vi "Robot Arm Sally Port.vi"(7 "Start Sally Port":bool, 8 "Abort":bool, 9 "Motor Speed":dbl=-0.2, 10 "Limit Switch Elbow":bool, 11 "Limit Switch Shoulder":bool) -> (0 "Done":bool=TRUE, 1 "Arcade Drive":cluster{"x":dbl, "y":dbl}, 2 "Set Elbow":dbl, 3 "Set Shoulder":dbl, 4 "Turn Arm":bool)   [LabVIEW 2015]
uses:
  sally_port_auto_states.ctl
  Sensors.vi
panel:
  in  "Kd":dbl=0.005
  in  "Kp":dbl=0.05
  in  "Ki":dbl
  in  "Drive Time":dbl=1.1
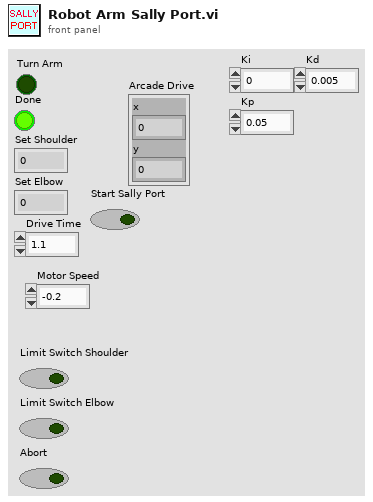
[diagram p1: front panel]
types:
  T1 = typedef "sally_port_auto_states.ctl" = enum16{"Ready", "Arm over", "Arm hook", "Arm rotate", "Move Forward for a bit", "drive thorugh", "Arm to rest", "stop"}
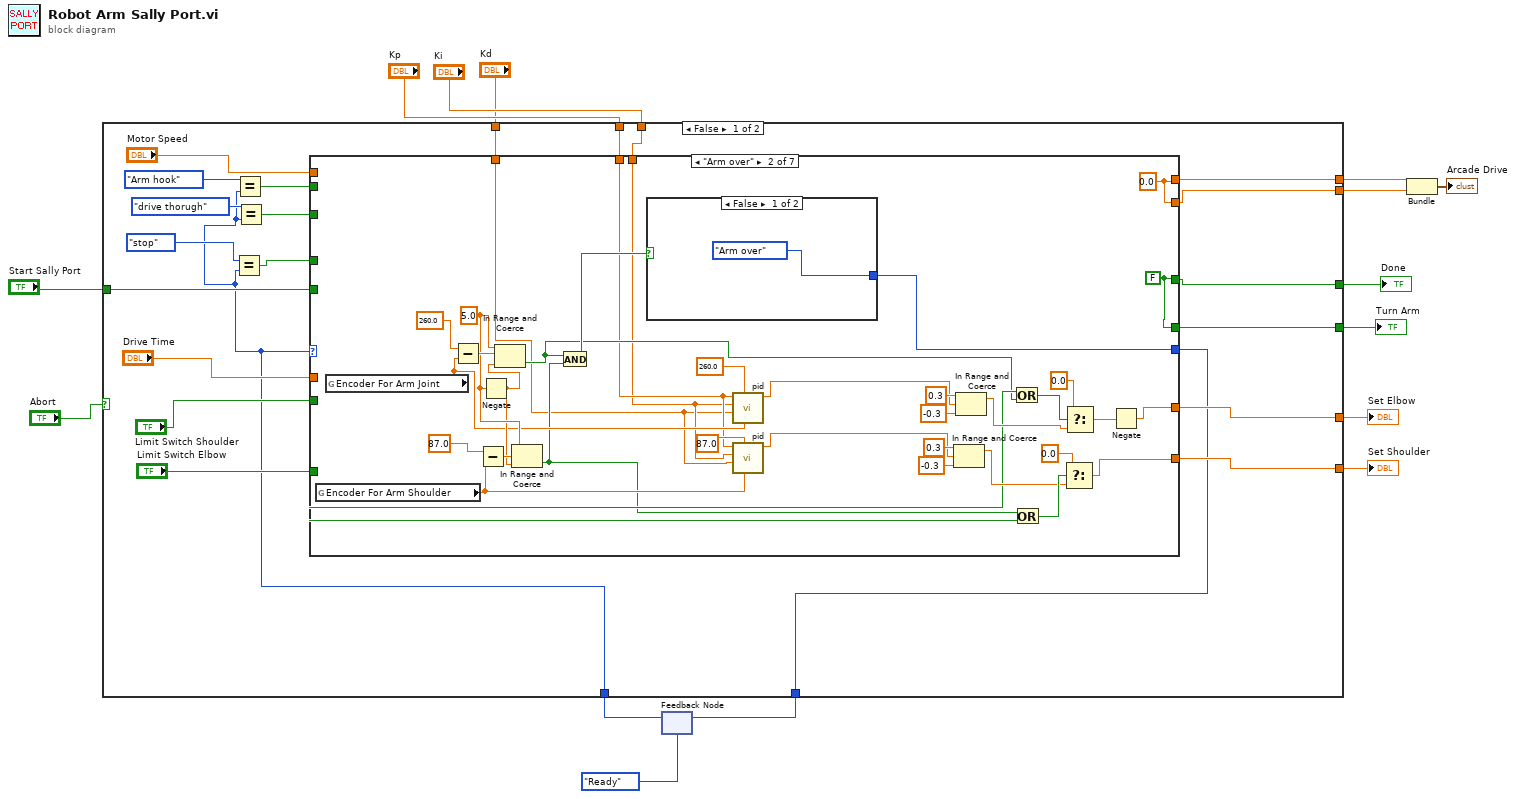
[diagram p0: block diagram]
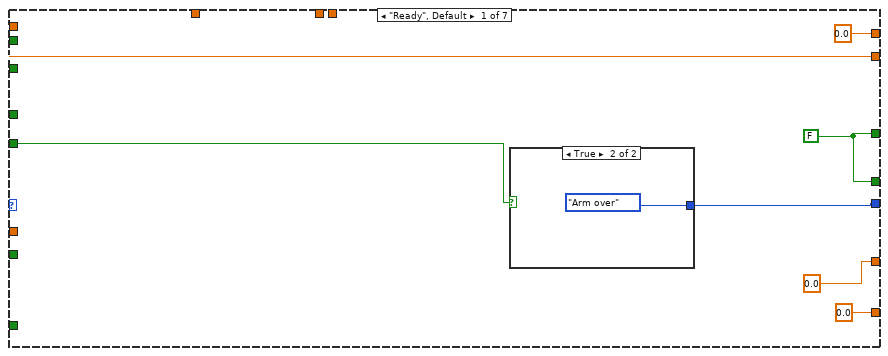
[diagram p2: hidden frame]
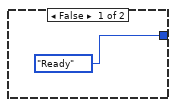
[diagram p3: hidden frame]
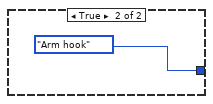
[diagram p4: hidden frame]
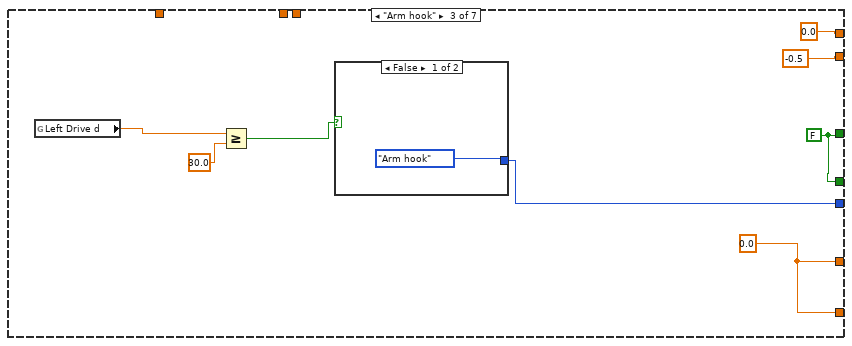
[diagram p5: hidden frame]
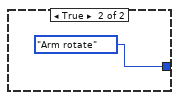
[diagram p6: hidden frame]
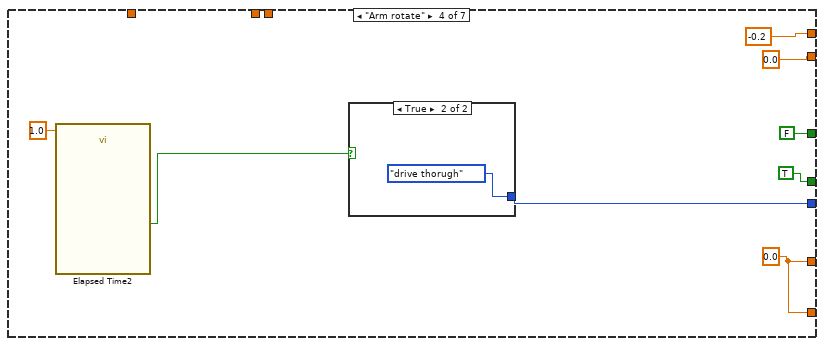
[diagram p7: hidden frame]
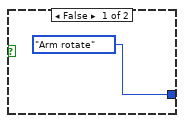
[diagram p8: hidden frame]
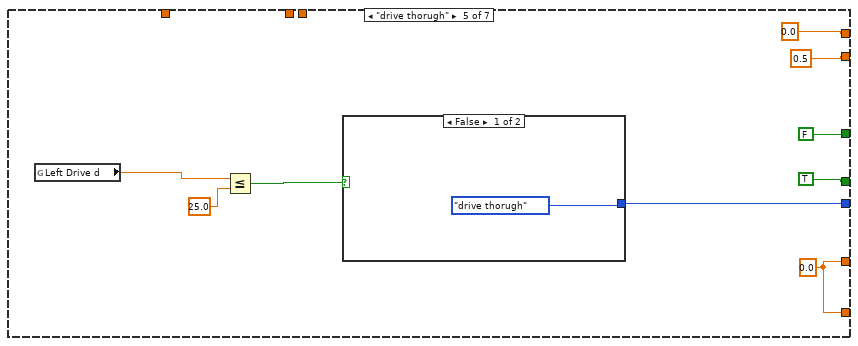
[diagram p9: hidden frame]
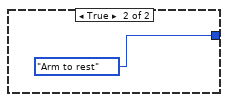
[diagram p10: hidden frame]
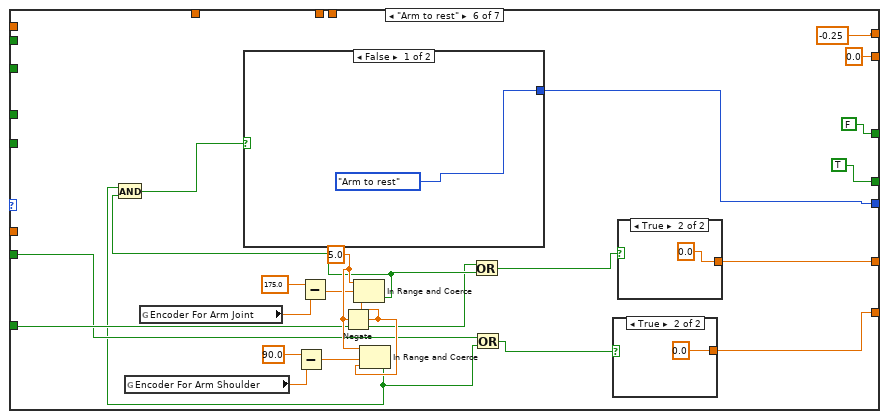
[diagram p11: hidden frame]
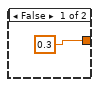
[diagram p12: hidden frame]
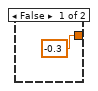
[diagram p13: hidden frame]
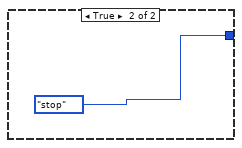
[diagram p14: hidden frame]
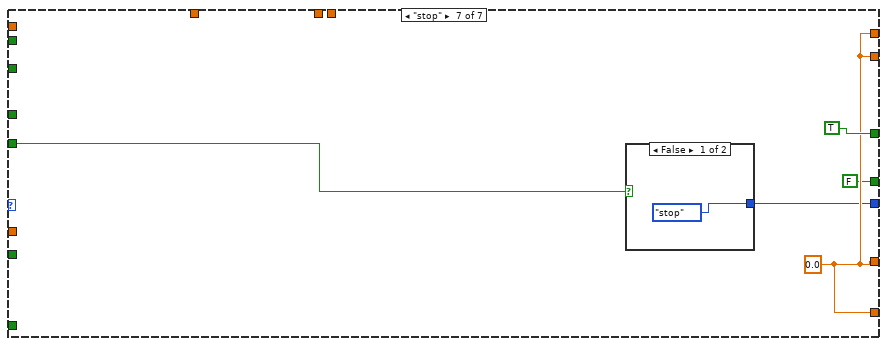
[diagram p15: hidden frame]
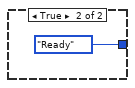
[diagram p16: hidden frame]
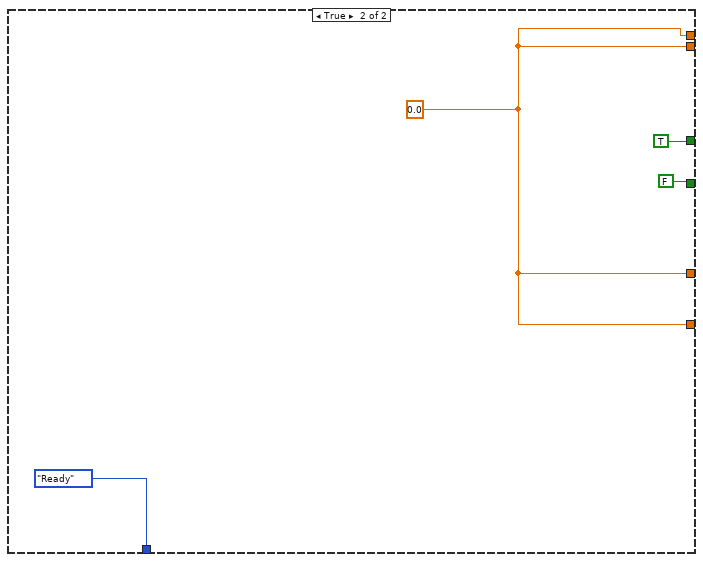
[diagram p17: hidden frame]
diagram:
  n1 = feedback #1(sally_port_auto_states."Ready") -> (w7:T1)
  n2 = case shown="False" "Abort" {
    tunnel: [w33 w154] -> w15
    tunnel: [w32 w154] -> w14
    tunnel: [w31 TRUE] -> w13
    tunnel: [w30 w154] -> w12
    tunnel: [w29 w154] -> w11
    tunnel: [w28 FALSE] -> w9
    tunnel: w7 -> [w18 _]
    tunnel: [w27 sally_port_auto_states."Ready"] -> w6
    tunnel: "Kp" -> [w26 _]
    tunnel: "Ki" -> [w25 _]
    tunnel: "Kd" -> [w24 _]
    tunnel: "Start Sally Port" -> [w23 _]
    frame False {
      n3 = Equal?(x=sally_port_auto_states."stop", y=w18) -> (x = y?=w21:bool)
      n4 = Equal?(x=sally_port_auto_states."Arm hook", y=w18) -> (x = y?=w16:bool)
      n5 = Equal?(x=sally_port_auto_states."drive thorugh", y=w18) -> (x = y?=w20:bool)
      n6 = case shown="\"Arm over\"" w18 {
        tunnel: "Motor Speed" -> [w44 _ _ _ _ _ _]
        tunnel: "Drive Time" -> [_ _ _ _ _ _ _]
        tunnel: [0.0 w71 0.0 -0.2 0.0 -0.25 w147] -> w33
        tunnel: [w38 w47 w88 FALSE FALSE FALSE TRUE] -> w31
        tunnel: [0.0 ("Set Motor at S") w56 w91 w101 w110 w134 w147] -> w30
        tunnel: [0.0 ("Set Motor at 1") w55 w91 w101 w110 w135 w147] -> w29
        tunnel: [w44 w71 -0.5 0.0 0.5 0.0 ("Motor Speed") w147] -> w32
        tunnel: "Limit Switch Shoulder" -> [_ w54 _ _ _ w120 _]
        tunnel: "Limit Switch Elbow" -> [_ w53 _ _ _ w121 _]
        tunnel: [w40 w70 w92 w102 w111 w133 w146] -> w27
        tunnel: [w38 w47 w88 TRUE TRUE TRUE FALSE] -> w28
        tunnel: w23 -> [w39 _ _ _ _ _ w144]
        tunnel: w26 -> [_ w50 _ _ _ _ _]
        tunnel: w25 -> [_ w49 _ _ _ _ _]
        tunnel: w24 -> [_ w48 _ _ _ _ _]
        tunnel: w21 -> [_ _ _ _ _ _ _]
        tunnel: w20 -> [_ _ _ _ _ _ _]
        tunnel: w16 -> [_ _ _ _ _ _ _]
        frame "Ready", Default {
          w38 = FALSE
          n7 = case shown="True" w39 {
            tunnel: [sally_port_auto_states."Ready" sally_port_auto_states."Arm over"] -> w40
            frame False {
            }
            frame True {
            }
          }
        }
        frame "Arm over" {
          w75 = 5.0
          w47 = FALSE
          w71 = 0.0
          n8 = global read "Sensors.vi" "Encoder For Arm Shoulder"() -> (w73:dbl)
          n9 = global read "Sensors.vi" "Encoder For Arm Joint"() -> (w72:dbl)
          n10 = Subtract(x=260.0 ("setpoint"), y=w72) -> (x-y=w77:dbl)
          n11 = Subtract(x=87.0 ("setpoint"), y=w73) -> (x-y=w80:dbl)
          n12 = Negate(x=w75) -> (-x=w74:dbl)
          n13 = In Range and Coerce(upper limit=w75, x=w77, lower limit=w74) -> (In Range?=w52:bool)  [unwired: 1 out]
          n14 = In Range and Coerce(upper limit=w75, x=w80, lower limit=w74) -> (In Range?=w51:bool)  [unwired: 1 out]
          n15 = And(x=w52, y=w51) -> (x .and. y?=w78:bool)
          n16 = case shown="False" w78 {
            tunnel: [sally_port_auto_states."Arm over" sally_port_auto_states."Arm hook"] -> w70
            frame False {
            }
            frame True {
            }
          }
          n17 = call "pid.vi"("y"=w72, "setpoint"=260.0, "kd"=w48, "ki"=w49, "kp"=w50) -> ("Motor Command"=w61:dbl)  [unwired: 6 in]
          n18 = call "pid.vi"("y"=w73, "setpoint"=87.0, "kd"=w48, "ki"=w49, "kp"=w50) -> ("Motor Command"=w60:dbl)  [unwired: 6 in]
          n19 = In Range and Coerce(upper limit=0.3, x=w60, lower limit=-0.3) -> (coerced(x)=w59:dbl)  [unwired: 1 out]
          n20 = In Range and Coerce(upper limit=0.3, x=w61, lower limit=-0.3) -> (coerced(x)=w58:dbl)  [unwired: 1 out]
          n21 = Or(x=w53, y=w52) -> (x .or. y?=w62:bool)
          n22 = Or(x=w51, y=w54) -> (x .or. y?=w63:bool)
          n23 = Select(t=0.0, s=w63, f=w59) -> (s? t:f=w55:dbl)
          n24 = Select(t=0.0, s=w62, f=w58) -> (s? t:f=w57:dbl)
          n25 = Negate(x=w57) -> (-x=w56:dbl)
        }
        frame "Arm hook" {
          w91 = 0.0
          w88 = FALSE
          n26 = global read "Sensors.vi" "Left Drive d"() -> (w85:dbl)
          n27 = Greater Or Equal?(x=w85, y=30.0) -> (x >= y?=w86:bool)
          n28 = case shown="False" w86 {
            tunnel: [sally_port_auto_states."Arm hook" sally_port_auto_states."Arm rotate"] -> w92
            frame False {
            }
            frame True {
            }
          }
        }
        frame "Arm rotate" {
          w101 = 0.0
          n29 = call "Elapsed Time2"("Time Target (s)"=1.0) -> ("Time has Elapsed"=w98:bool)  [unwired: 11 in, 7 out]
          n30 = case shown="True" w98 {
            tunnel: [sally_port_auto_states."Arm rotate" sally_port_auto_states."drive thorugh"] -> w102
            frame False {
            }
            frame True {
            }
          }
        }
        frame "drive thorugh" {
          w110 = 0.0
          n31 = global read "Sensors.vi" "Left Drive d"() -> (w106:dbl)
          n32 = Less Or Equal?(x=w106, y=25.0) -> (x <= y?=w105:bool)
          n33 = case shown="False" w105 {
            tunnel: [sally_port_auto_states."drive thorugh" sally_port_auto_states."Arm to rest"] -> w111
            frame False {
            }
            frame True {
            }
          }
        }
        frame "Arm to rest" {
          w130 = 5.0
          n34 = global read "Sensors.vi" "Encoder For Arm Shoulder"() -> (w126:dbl)
          n35 = global read "Sensors.vi" "Encoder For Arm Joint"() -> (w125:dbl)
          n36 = Subtract(x=90.0, y=w126) -> (x-y=w129:dbl)
          n37 = Subtract(x=175.0, y=w125) -> (x-y=w128:dbl)
          n38 = Negate(x=w130) -> (-x=w131:dbl)
          n39 = In Range and Coerce(upper limit=w130, x=w128, lower limit=w131) -> (In Range?=w123:bool)  [unwired: 1 out]
          n40 = In Range and Coerce(upper limit=w130, x=w129, lower limit=w131) -> (In Range?=w119:bool)  [unwired: 1 out]
          n41 = And(x=w119, y=w123) -> (x .and. y?=w136:bool)
          n42 = case shown="False" w136 {
            tunnel: [sally_port_auto_states."Arm to rest" sally_port_auto_states."stop"] -> w133
            frame False {
            }
            frame True {
            }
          }
          n43 = Or(x=w121, y=w123) -> (x .or. y?=w122:bool)
          n44 = Or(x=w120, y=w119) -> (x .or. y?=w118:bool)
          n45 = case shown="True" w118 {
            tunnel: [-0.3 0.0] -> w135
            frame False {
            }
            frame True {
            }
          }
          n46 = case shown="True" w122 {
            tunnel: [0.3 0.0] -> w134
            frame False {
            }
            frame True {
            }
          }
        }
        frame "stop" {
          w147 = 0.0
          n47 = case shown="False" w144 {
            tunnel: [sally_port_auto_states."stop" sally_port_auto_states."Ready"] -> w146
            frame False {
            }
            frame True {
            }
          }
        }
      }
    }
    frame True {
      w154 = 0.0
    }
  }
  "Done" <- w13
  "Set Elbow" <- w12
  "Set Shoulder" <- w11
  "Turn Arm" <- w9
  n48 = feedback-in #1(w6) -> ()
  n49 = Bundle(w15, "Motor Speed"=w14) -> (→"Arcade Drive":cluster{dbl, "Motor Speed":dbl})  [unwired: 1 in]
